vi "uTTA_LogSerial.vi"(4 "error in":errorcluster, 6 "Data_Sent":string) -> (0 "error out":errorcluster)   [LabVIEW 2021]
uses:
  uTTA_GV_Serial_Monitor.vi
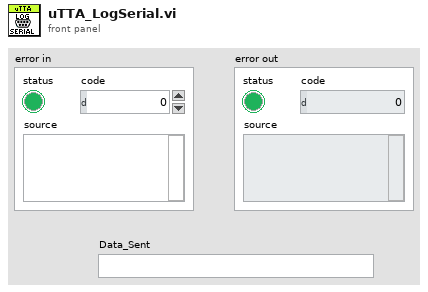
[diagram p1: front panel]
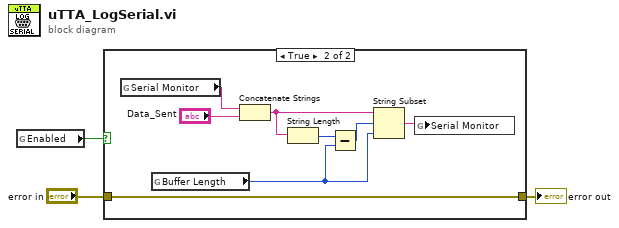
[diagram p0: block diagram]
diagram:
  n1 = global read "uTTA_GV_Serial_Monitor.vi" "Enabled"() -> (w3:bool)
  n2 = case shown="True" w3 {
    tunnel: "error in" -> [w4 w5]
    tunnel: [w4 w5] -> w1
    frame False {
    }
    frame True {
      n3 = global read "uTTA_GV_Serial_Monitor.vi" "Serial Monitor"() -> (w11:string)
      n4 = global read "uTTA_GV_Serial_Monitor.vi" "Buffer Length"() -> (w7:u32)
      n5 = Concatenate Strings(w11, "Data_Sent") -> (w9:string)
      n6 = String Length(string=w9) -> (length=w8:i32)
      n7 = Subtract(x=w8, y=w7) -> (x-y=w6:u32)
      n8 = String Subset(string=w9, offset (0)=w6, length (rest)=w7) -> (substring=w12:string)
      n9 = global write "uTTA_GV_Serial_Monitor.vi" "Serial Monitor"(w12) -> ()
    }
  }
  "error out" <- w1
